vi "get&set Size.vi"(6 "Get/Set? (Set)":bool=TRUE, 8 "error in (no error)":errorcluster, 10 "3D Size":T1, 11 "VGS_VolumeDescriptor+File in":refnum<class "VGS_VolumeDescriptor+File.lvclass">) -> (0 "error out":errorcluster, 2 "3D Size":T1, 3 "VGS_VolumeDescriptor+File out":refnum<class "VGS_VolumeDescriptor+File.lvclass">)   [LabVIEW 2022 SP3, in "LV_VGS.lvlib" / "VGS_VolumeDescriptor+File.lvclass"]
doc: "<B>Defines physical position of a single slice file. </B>\n\nDefines the relative physical position of a single slice file. Use this function if the file represents a single xy-slice (z-size is 1).\n\nThis function is equivalent to calling setPositionList() with a list of size 1. See setPositionList() for details. \n\n<B>bool VGS::Project::Interop::VolumeDescriptor::File::setPositionList ( List< float >^ positionList ) </B>\n\nDefines physical positions of the file's slices. \n\nDefines the relative physical position of all the slices represented by this file. Use this function to define non-equidistant slices: normally, the slice distance is determined globally by the z-component of VolumeDescriptor.Resolution, i.e. all given xy-slices are the same distance apart. If your scanned data has varying slice distances, however, you can define a kind of physical position (in mm) for each slice. These distances will then be used instead of the z-resolution value, which will be ignored.\n\n You cannot \"mix\" specifications: if you specify a position list, you must do it for all files in the VolumeDescriptor, and each file must specify as many positions as its z-size indicates! \n Optional definition. The default value is an empty list."
uses:
  VGS_VolumeDescriptor+File.lvclass
  typedefs/3D Size (I32).ctl
  VGS_VolumeDescriptor+File.lvclass/VGS_VolumeDescriptor+File.ctl
  C:/Users/Andrey/Documents/GitHub/LV_VGS/vgs_project.dll
  vgs_project.dll
  LV_VGS.lvlib
panel:
  # "-Set\n-Get"
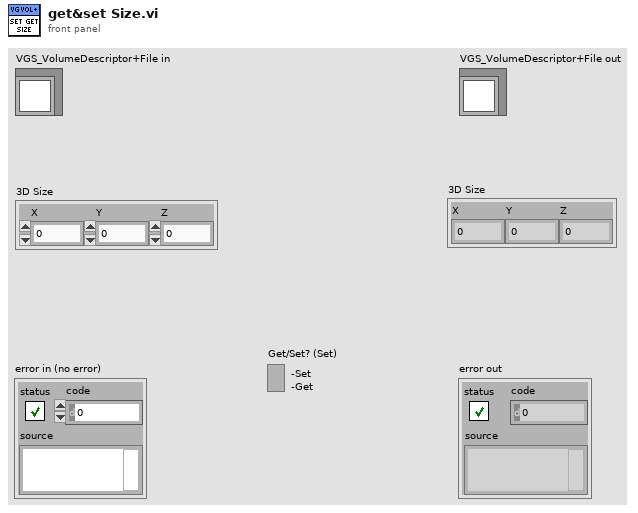
[diagram p1: front panel]
types:
  T1 = typedef "LV_VGS.lvlib/3D Size (I32).ctl" = cluster{"X":i32, "Y":i32, "Z":i32}
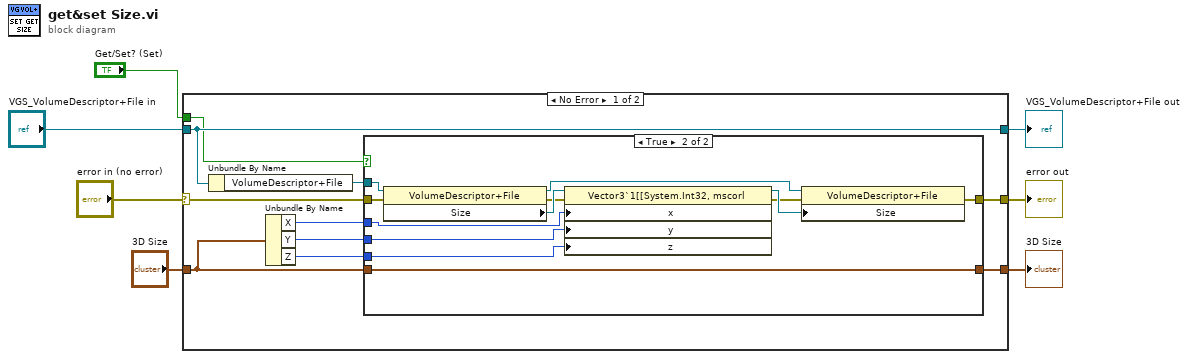
[diagram p0: block diagram]
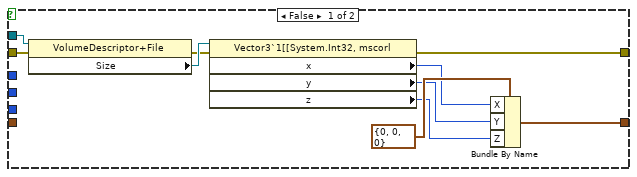
[diagram p2: hidden frame]
diagram:
  n1 = case shown="No Error" "error in (no error)" {
    selector: "error in (no error)" -> [w15 w42]
    tunnel: [w14 w42] -> w6
    tunnel: [w17 w41] -> w4
    tunnel: "VGS_VolumeDescriptor+File in" -> [w17 w41]
    tunnel: "Get/Set? (Set)" -> [w13 _]
    tunnel: [w12 w40] -> w1
    tunnel: "3D Size" -> [w8 w40]
    frame No Error {
      n2 = Unbundle By Name(w17) -> ("VolumeDescriptor+File"=w16:refnum<k24>)
      n3 = Unbundle By Name(w8) -> ("X"=w11:i32, "Y"=w10:i32, "Z"=w9:i32)
      n4 = case shown="True" w13 {
        tunnel: w16 -> [w27 w32]
        tunnel: w15 -> [w26 w30]
        tunnel: [w18 w33] -> w14
        tunnel: w8 -> [_ w39]
        tunnel: [w20 w39] -> w12
        tunnel: w11 -> [_ w38]
        tunnel: w10 -> [_ w37]
        tunnel: w9 -> [_ w36]
        frame False {
          n5 = property class="VolumeDescriptor+File"(reference=w27, error in=w26) -> (error out=w19:errorcluster, "Size"=w25:refnum<k24>)  [unwired: 1 out]
          n6 = property class="Vector3`1[[System.Int32, mscorl"(reference=w25, error in=w19) -> (error out=w18:errorcluster, "x"=w23:i32, "y"=w22:i32, "z"=w21:i32)  [unwired: 1 out]
          n7 = Bundle By Name(cluster=T1 {"X"=0, "Y"=0, "Z"=0} ("3D Size"), "X"=w23, "Y"=w22, "Z"=w21) -> (w20:T1)
        }
        frame True {
          n8 = property class="VolumeDescriptor+File"(reference=w32, error in=w30) -> (reference out=w28:refnum<k24>, error out=w29:errorcluster, "Size"=w31:refnum<k24>)
          n9 = property class="Vector3`1[[System.Int32, mscorl"(reference=w31, error in=w29, "x"=w38, "y"=w37, "z"=w36) -> (reference out=w35:refnum<k24>, error out=w34:errorcluster)
          n10 = property class="VolumeDescriptor+File"(reference=w28, error in=w34, "Size"=w35) -> (error out=w33:errorcluster)  [unwired: 1 out]
        }
      }
    }
    frame Error {
    }
  }
  "error out" <- w6
  "VGS_VolumeDescriptor+File out" <- w4
  "3D Size" <- w1
